vi "test_fast_PID_chain2.vi"() -> ()   [LabVIEW 2013]
uses:
  <vilib>/measure/NI_MABase.lvlib
  Scope5782/Scope/controls/Memory block.ctl
panel:
  out "Waveform Graph 4":i16[](graph)
  out "Waveform Graph 3":dbl[][](graph)
  out "Waveform Graph 2":i16[](graph)
  out "Waveform Graph":dbl[](graph)
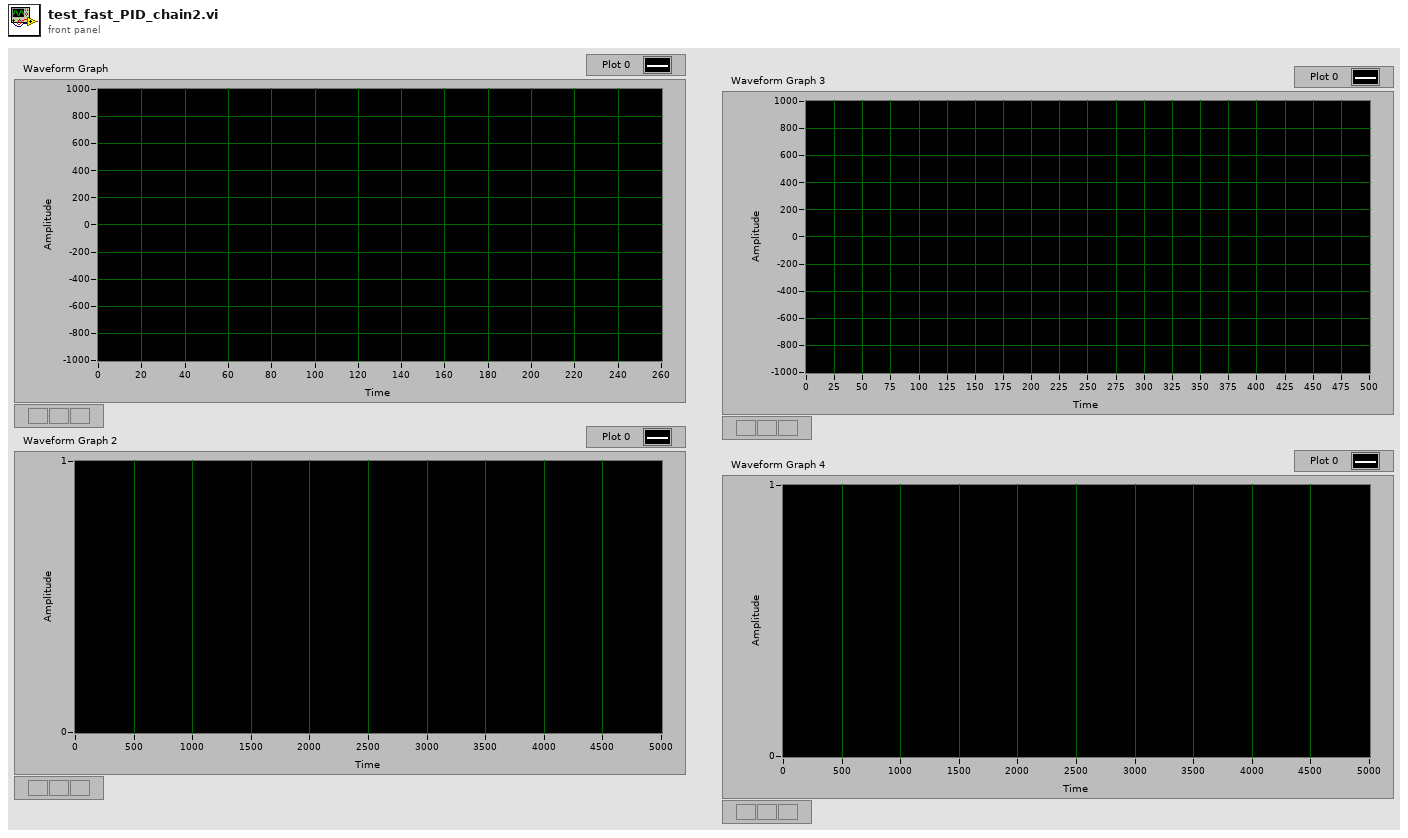
[diagram p1: front panel]
types:
  T1 = typedef "Memory block.ctl" = enum16{"Setpoint", "Beam"}
  T2 = cluster{"frequency":dbl, "amplitude":dbl, "phase":dbl}[]
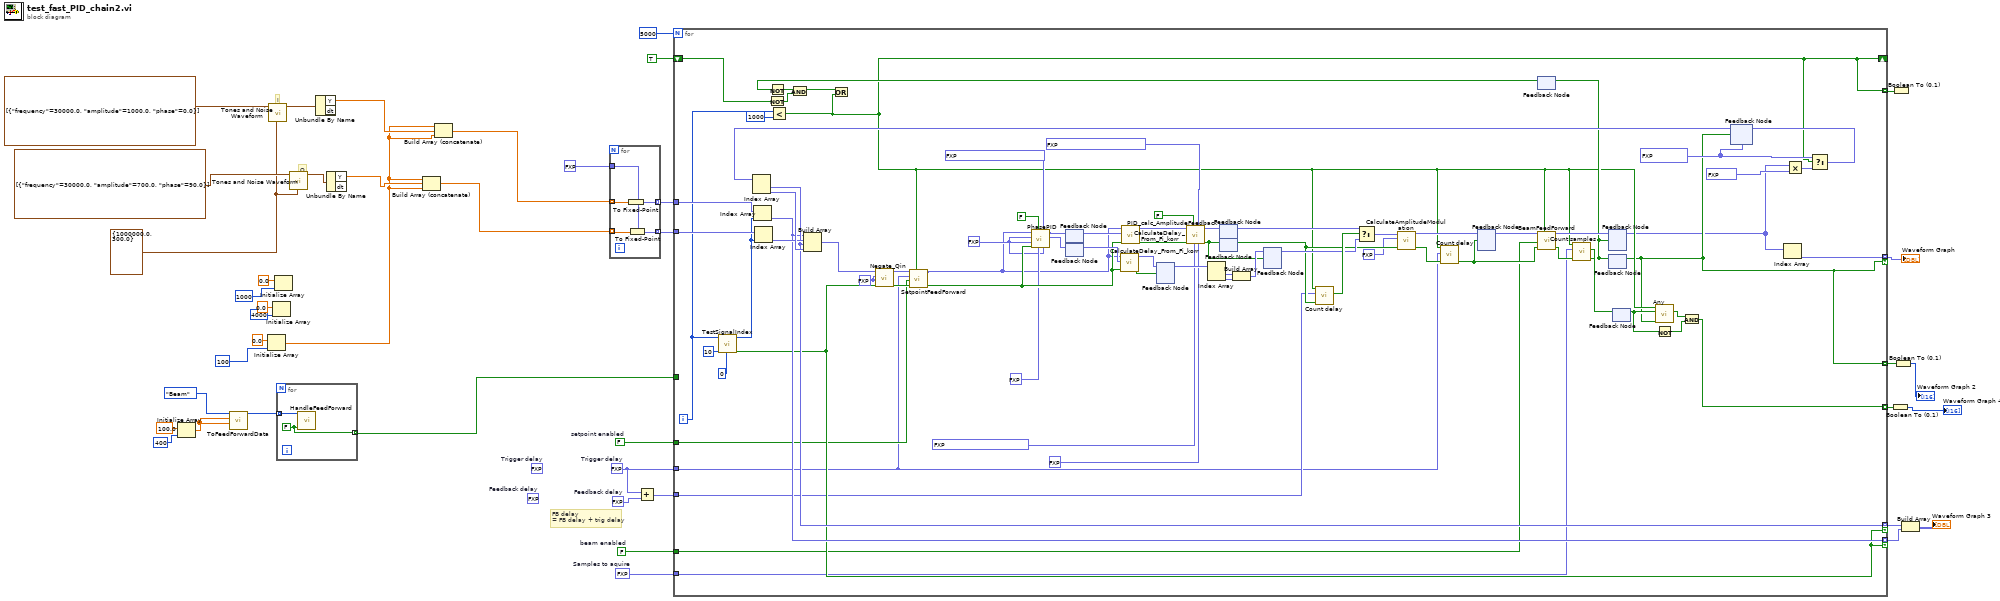
[diagram p0: block diagram]
diagram:
  (unwired) fxp<+/-,16,16> 10.0  # Feedback delay
  (unwired) fxp<+/-,16,16> 25.0  # Trigger delay
  w31 = FALSE  # beam enabled
  w32 = fxp<+,16,16> 250.0  # Samples to aquire
  w33 = FALSE  # setpoint enabled
  w36 = fxp<+/-,16,16> 0.0  # Feedback delay
  w34 = fxp<+/-,16,16> 0.0  # Trigger delay
  w29 = cluster{"Fs":dbl, "#s":dbl} {"Fs"=1000000.0, "#s"=300.0} ("sampling info")
  # "Q"
  # "I"
  # "FB delay\n= FB delay + trig delay"
  n1 = Initialize Array(100.0 ("element"), 400 ("dimension size")) -> (w8:dbl[])
  n2 = call "ToFeedForwardData.vi"("values Q"=w8, "values I"=w8, "Memory block"=Memory_block."Beam") -> ("Data"=w12:u64[])  [unwired: 8 in]
  n3 = Initialize Array(0.0 ("element"), 100 ("dimension size")) -> (w19:dbl[])
  n4 = call <vilib>:"Tones and Noise Waveform.vi"("sampling info"=w29, "tones"=T2 [{"frequency"=30000.0, "amplitude"=1000.0, "phase"=0.0}]) -> ("signal out"=w40:waveform(dbl))  [unwired: 8 in, 1 out]
  n5 = Initialize Array(0.0 ("element"), 4000 ("dimension size")) -> ()  [unwired: 1 out]
  n6 = Initialize Array(0.0 ("element"), 1000 ("dimension size")) -> ()  [unwired: 1 out]
  n7 = for {
    tunnel: w12 -> [w44] mode=indexing
    tunnel: [w43] -> w5 mode=indexing
    w43 = FALSE ("timed out")
    n8 = call "HandleFeedForward.vi"("timed out"=w43, "Value"=w44) -> ()  [unwired: 10 in]
  }
  n9 = call <vilib>:"Tones and Noise Waveform.vi"("sampling info"=w29, "tones"=T2 [{"frequency"=30000.0, "amplitude"=700.0, "phase"=90.0}]) -> ("signal out"=w26:waveform(dbl))  [unwired: 8 in, 1 out]
  n10 = Unbundle By Name(w40) -> ("Y"=w22:dbl[])  [unwired: 1 out]
  n11 = Unbundle By Name(w26) -> ("Y"=w21:dbl[])  [unwired: 1 out]
  n12 = Build Array (concatenate)(w19, w21, w19) -> (w18:dbl[])
  n13 = Build Array (concatenate)(w19, w22, w19) -> (w13:dbl[])
  n14 = for {
    tunnel: w18 -> [w48] mode=indexing
    tunnel: fxp<+/-,16,14> 0.0 ("fixed-point type") -> [w49]
    tunnel: [w47] -> w39 mode=indexing
    tunnel: w13 -> [w45] mode=indexing
    tunnel: [w46] -> w17 mode=indexing
    n15 = To Fixed-Point(number=w45) -> (fixed-point=w46:fxp<+/-,16,14>)  [unwired: 1 in]
    n16 = To Fixed-Point(fixed-point type=w49, number=w48) -> (fixed-point=w47:fxp<+/-,16,14>)
  }
  n17 = Add(x=w34, y=w36) -> (x+y=w35:fxp<+/-,17,17>)
  n18 = for {
    N: 5000 -> [_]
    tunnel: w39 -> [w124]
    tunnel: [w54] -> w38 mode=indexing
    tunnel: [w123] -> w1 mode=indexing if=w54
    tunnel: w35 -> [w62]
    tunnel: w34 -> [w61]
    tunnel: w33 -> [w63]
    tunnel: w32 -> [w60]
    tunnel: w31 -> [w58]
    tunnel: w17 -> [w122]
    shift-right: [w56] -> _
    shift-left: TRUE -> [w115]
    tunnel: [w56] -> w14 mode=indexing
    tunnel: [w106] -> w7 mode=indexing if=w71
    tunnel: [w105] -> w6 mode=indexing if=w71
    tunnel: w5 -> [_]
    tunnel: [w55] -> w4 mode=indexing
    i -> [w118]
    w64 = fxp<+/-,16,14> 0.0 ("DC offset chan 1")
    w107 = fxp<+/-,21,13>[] [0.0, 0.0]
    w67 = fxp<+/-,32,4> 0.0 ("Fi_start")
    n19 = call "TestSignalIndex.vi"("initial delay"=0, "cycles per sample"=10, "index"=w118) -> ("valid out"=w71:bool, "array index"=w110:i32)  [unwired: 7 in]
    n20 = Index Array(array=w122, index=w110) -> (element=w105:fxp<+/-,16,14>)
    n21 = Index Array(array=w124, index=w110) -> (element=w111:fxp<+/-,16,14>)
    n22 = Not(x=w115) -> (.not. x?=w113:bool)
    n23 = Less?(x=w118, y=1000) -> (x < y?=w56:bool)
    n24 = feedback #1() -> (w99:fxp<+/-,32,4>)  [unwired: 1 in]
    n25 = feedback #2() -> (w101:fxp<+/-,32,4>)  [unwired: 1 in]
    n26 = feedback #3() -> (w90:fxp<+/-,16,14>[])  [unwired: 1 in]
    n27 = Index Array(array=w90) -> (element #1=w92:fxp<+/-,16,14>, element #2=w91:fxp<+/-,16,14>)  [unwired: 2 in]
    n28 = feedback #4() -> (w94:fxp<+/-,16,14>[])  [unwired: 1 in]
    n29 = feedback #5() -> (w95:bool)  [unwired: 1 in]
    n30 = Build Array(w92, w91) -> (w89:fxp<+/-,16,14>[])
    n31 = feedback #6() -> (w96:fxp<+/-,16,14>[])  [unwired: 1 in]
    n32 = call "Count delay.vi"("input valid"=w95, "Count to skip"=w62, "Reset"=w56) -> ("count done?"=w97:bool)  [unwired: 7 in, 1 out]
    n33 = Select(t=w94, s=w97, f=w96) -> (s? t:f=w93:fxp<+/-,16,14>[])
    n34 = call "CalculateAmplitudeModulation.vi"("input valid"=w95, "AM_factor"=fxp<+/-,16,2> 1.0, "Data in"=w93) -> ("output valid"=w83:bool, "Data out"=w98:fxp<+/-,16,14>[])  [unwired: 7 in]
    n35 = call "Count delay.vi"("input valid"=w83, "Count to skip"=w61, "Reset"=w56) -> ("output valid"=w86:bool)  [unwired: 7 in, 1 out]
    n36 = feedback #7() -> (w88:fxp<+/-,16,14>[])  [unwired: 1 in]
    n37 = feedback-in #7(w98, w86) -> ()
    n38 = feedback #8() -> (w116:bool)  [unwired: 1 in]
    n39 = Not(x=w116) -> (.not. x?=w114:bool)
    n40 = And(x=w114, y=w113) -> (x .and. y?=w112:bool)
    n41 = Or(x=w112, y=w56) -> ()  [unwired: 1 out]
    n42 = call "BeamFeedForward.vi"("Reset"=w56, "input valid"=w86, "beam enabled"=w58, "Data in"=w88) -> ("output valid"=w77:bool, "Data out"=w87:fxp<+/-,16,14>[])  [unwired: 6 in]
    n43 = call "Count samples.vi"("input valid"=w77, "Samples to count"=w60, "Reset"=w56) -> ("output valid"=w57:bool, "counting"=w76:bool)  [unwired: 7 in]
    n44 = feedback-in #8(w57) -> ()
    n45 = feedback #9() -> (w53:fxp<+/-,16,14>[])  [unwired: 1 in]
    n46 = feedback-in #9(w87, w57) -> ()
    n47 = feedback #10() -> (w54:bool)  [unwired: 1 in]
    n48 = feedback-in #10(w57) -> ()
    n49 = feedback #11() -> (w75:bool)  [unwired: 1 in]
    n50 = feedback-in #11(w76) -> ()
    n51 = call "Any.vi"("input valid"=w54, "Value"=w75, "Reset"=w56) -> ("Any?"=w74:bool)  [unwired: 7 in, 1 out]
    n52 = Not(x=w75) -> (.not. x?=w73:bool)
    n53 = And(x=w74, y=w73) -> (x .and. y?=w55:bool)
    n54 = feedback #12(w107) -> (w120:fxp<+/-,21,13>[])
    n55 = Index Array(array=w120) -> (element #1=w106:fxp<+/-,21,13>, element #2=w119:fxp<+/-,21,13>)  [unwired: 2 in]
    n56 = Build Array(w105, w111, w106, w119) -> (w72:fxp<+/-,22,14>[])
    n57 = call "Negate_Qin.vi"("valid in"=w71, "DC offset chan 1"=w64, "DC offset chan 0"=w64, "Data in"=w72) -> ("valid out"=w102:bool, "Data out"=w52:fxp<+/-,16,14>[])  [unwired: 6 in]
    n58 = call "SetpointFeedForward.vi"("Reset"=w56, "input valid"=w102, "setpoint enabled"=w63, "Samples to skip"=w61, "Data in"=w52) -> ("output valid"=w100:bool, "Data out"=w51:fxp<+/-,16,14>[])  [unwired: 5 in]
    n59 = call "PhasePID.vi"("Kd/Tau"=w67, "Ki*Tau"=fxp<+/-,32,4> 0.0010000020265579224, "Kp"=fxp<+/-,32,4> 0.0, "Reset"=FALSE, "input valid"=w100, "Fi_delta"=w67, "Fi_start"=w67, "Data in"=w51) -> ("Fi_korr"=w103:fxp<+/-,32,4>, "Fi_korr PID"=w104:fxp<+/-,32,4>)  [unwired: 1 in, 1 out]
    n60 = feedback-in #1(w104) -> ()
    n61 = feedback-in #2(w103) -> ()
    n62 = call "CalculateDelay_From_Fi_korr.vi"("input valid"=w100, "fi_korr"=w101, "Data in"=w51) -> ("output valid"=w81:bool, "Data out"=w80:fxp<+/-,16,14>[])  [unwired: 7 in]
    n63 = call "CalculateDelay_From_Fi_korr.vi"("input valid"=w100, "fi_korr"=w99, "Data in"=w51) -> ("output valid"=w79:bool, "Data out"=w78:fxp<+/-,16,14>[])  [unwired: 7 in]
    n64 = feedback-in #3(w80, w81) -> ()
    n65 = call "PID_calc_AmplitudeFeedback.vi"("Kd/Tau"=fxp<+/-,32,6> 0.0 ("Data"), "Ki*Tau"=fxp<+/-,32,6> 0.0010000020265579224 ("Data"), "Kp"=fxp<+/-,32,6> 0.010000020265579224 ("Data"), "Enabled"=FALSE, "input valid"=w79, "Data in"=w78) -> ("output valid"=w84:bool, "data out"=w85:fxp<+/-,16,14>[])  [unwired: 2 in, 2 out]
    n66 = feedback-in #4(w85) -> ()
    n67 = feedback-in #5(w84) -> ()
    n68 = feedback-in #6(w89, w84) -> ()
    n69 = Index Array(array=w53) -> (element=w123:fxp<+/-,16,14>)  [unwired: 1 in]
    n70 = Multiply(x=w53, y=fxp<+,5,-1> 0.296875 ("Q out")) -> (x*y=w109:fxp<+/-,21,13>[])
    n71 = Select(t=w107, s=w56, f=w109) -> (s? t:f=w108:fxp<+/-,21,13>[])
    n72 = feedback-in #12(w108, w54) -> ()
  }
  "Waveform Graph" <- w1
  n73 = Boolean To (0,1)(Boolean=w4) -> (0, 1=→"Waveform Graph 4":i16[])
  n74 = Boolean To (0,1)(Boolean=w14) -> ()  [unwired: 1 out]
  n75 = Boolean To (0,1)(Boolean=w38) -> (0, 1=→"Waveform Graph 2":i16[])
  n76 = Build Array(w7, w6) -> (→"Waveform Graph 3":fxp<+/-,22,14>[][])
